vi "testDBL.vi"() -> ()   [LabVIEW 2026]
panel:
  out "Waveform Graph":dbl[](graph)
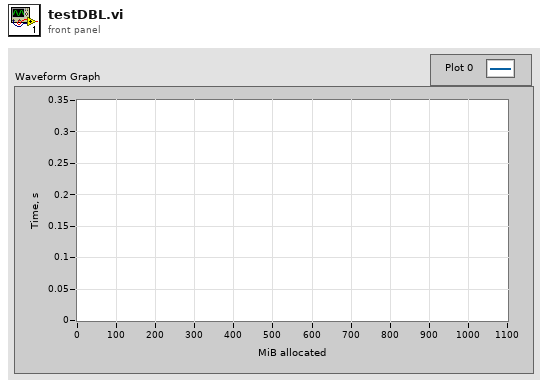
[diagram p1: front panel]
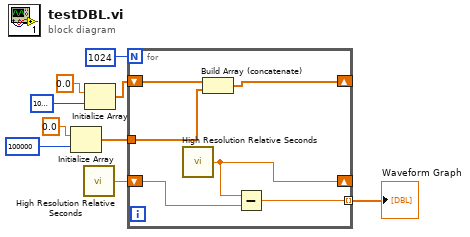
[diagram p0: block diagram]
diagram:
  n1 = Initialize Array(0.0 ("element"), 100000 ("dimension size")) -> (w1:dbl[])
  n2 = call <vilib>:"High Resolution Relative Seconds.vi"() -> ("relative seconds"=w5:dbl)
  n3 = Initialize Array(0.0 ("element"), 1048576 ("dimension size")) -> (w7:dbl[])
  n4 = for {
    N: 1024 -> [_]
    shift-right: [w14] -> _
    shift-left: w7 -> [w15]
    shift-right: [w11] -> _
    shift-left: w5 -> [w13]
    tunnel: [w12] -> w4 mode=indexing
    tunnel: w1 -> [w10]
    n5 = call <vilib>:"High Resolution Relative Seconds.vi"() -> ("relative seconds"=w11:dbl)
    n6 = Build Array (concatenate)(w15, w10) -> (w14:dbl[])
    n7 = Subtract(x=w11, y=w13) -> (x-y=w12:dbl)
  }
  "Waveform Graph" <- w4
